vi "Start and Stop Continuous.vi"() -> (0 "x*y 3":dbl)   [LabVIEW 2010]
panel:
  out "Pitch Gauge (Degrees) 2":dbl(slide) scale=-90.0..90.0
  out "Roll Gauge (Degrees) 3":dbl(knob) scale=-180.0..180.0
  out "Roll Gauge (Degrees) 2":dbl(knob) scale=-180.0..180.0
  out "x*y 2":dbl
  out "x*y":dbl
  out "Command String":string
  in  "stop":bool
  in  "Stop Continuous":bool
  in  "Start":bool
  in  "Baud Rate":u32=115200
  in  "Serial Port":refnum<visa-resource-name>="COM1"
  out "Error Output":errorcluster
  out "Acceleration (G's)":dbl[](array[numeric])
  # "HOW TO USE\n\nSelect the port that your sensor is connected to, then click the \"Run\" arrow.  Click \"Start Continuous\" to start continuous mode and \"Stop Continuous\"  to stop continuous mode. Press STOP to stop vi and close port. The Acceleration and Angular Rate (0xC2 command) is displayed. \n\nFor USB sensors, use the Windows Device Manager to determine which COM port has been assigned to your sensor.  Your device will be listed as a  \"MicroStrain Virtual COM Port\".\n\nThe default BAUD rate is 115200 on all devices.  \n\nIf your device's port does not appear in the serial port control  then try quitting and relaunching LabVIEW."
  # "This example uses the 0xC4 command to start the 3DM-GX3 sending 0xC2 data packets continuously.   The data rate may be changed by using the Set Data Rate example."
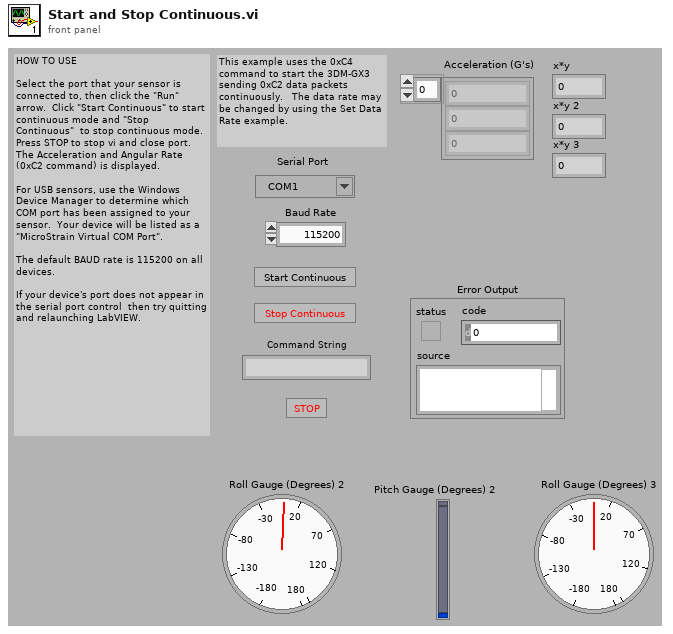
[diagram p1: front panel]
types:
  T1 = cluster{"Cmd/SOP Byte":string, "Header Size":u16, "Len":u16, "Chksum Start":u16, "Chksum End":i16, "InHdr":bool}[]
  T2 = cluster{"Command Byte":u8, "Acceleration Vector":cluster{sgl, sgl, sgl}, "Timer Ticks":u32, "Checksum":u16}
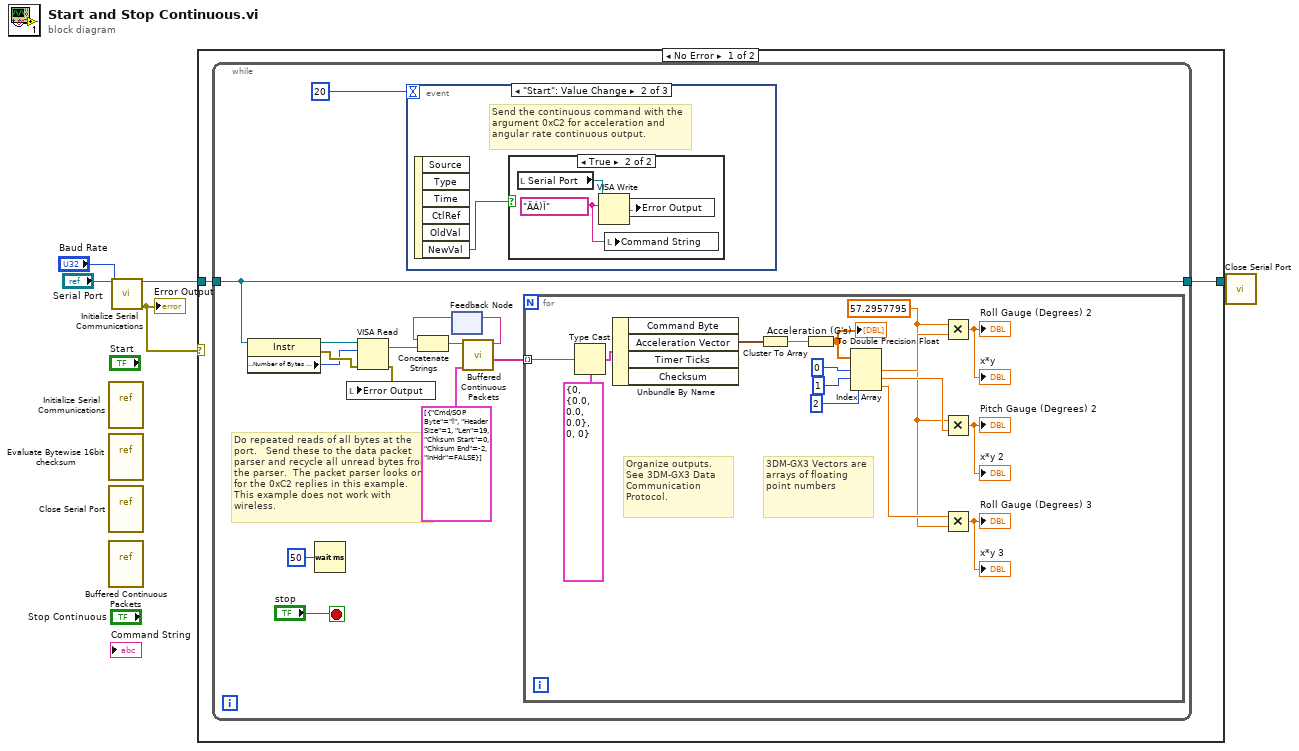
[diagram p0: block diagram]
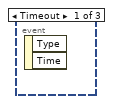
[diagram p2: hidden frame]
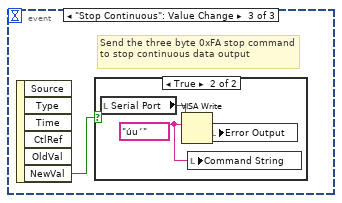
[diagram p4: hidden frame]
diagram:
  n1 = vi-ref "Initialize Serial Communications.vi"() -> ()  [unwired: 1 out]
  n2 = vi-ref "Evaluate Bytewise 16bit checksum.vi"() -> ()  [unwired: 1 out]
  n3 = vi-ref "Close Serial Port.vi"() -> ()  [unwired: 1 out]
  n4 = vi-ref "Buffered Continuous Packets.vi"() -> ()  [unwired: 1 out]
  n5 = call "Initialize Serial Communications.vi"("Serial Port"="Serial Port", "Baud Rate"="Baud Rate") -> ("Serial Port Out"=w3:refnum<visa-resource-name>, "error out"=w1:errorcluster)  [unwired: 12 in]
  "Error Output" <- w1
  n6 = case shown="No Error" w1 {
    tunnel: w3 -> [w7 w46]
    tunnel: [w6 w46] -> w2
    frame No Error {
      n7 = while {
        tunnel: w7 -> [w15]
        tunnel: [w15] -> w6
        stop <- "stop" stop-if-true
        # "Do repeated reads of all bytes at the port.   Send these to the data packet parser and recycle all unread bytes from the parser.  The packet parser looks only for the 0xC2 replies in this example.  This example does not work with wireless."
        n8 = property class="Instr"(reference=w15) -> (reference out=w18:refnum<visa-resource-name>, error out=w21:errorcluster, "Serial Settings:Number of Bytes at Serial Port"=w19:u32)  [unwired: 1 in]
        n9 = Wait (ms)(milliseconds to wait=u32 50) -> ()  [unwired: 1 out]
        n10 = VISA Read(VISA resource name=w18, byte count=w19, error in (no error)=w21) -> (read buffer=w20:string, error out=w14:errorcluster)  [unwired: 2 out]
        n11 = local write "Error Output"(w14) -> ()
        n12 = event shown="[1] \"Start\": Value Change" {
          selector: _ -> [_ _ _]
          dyn-events: _ -> [_ _ _]
          timeout: 20 -> [_ _ _]
          event Timeout {
            n13 = event-data() -> ()  [unwired: 1 in, 2 out]
          }
          event "Start": Value Change {
            # "Send the continuous command with the argument 0xC2 for acceleration and angular rate continuous output."
            n14 = event-data() -> ("NewVal"=w22:bool)  [unwired: 1 in, 5 out]
            n15 = case shown="True" w22 {
              frame False {
              }
              frame True {
                w23 = "ÄÁ)Î" ("write buffer")
                n16 = local read "Serial Port"() -> (w25:refnum<visa-resource-name>)
                n17 = VISA Write(VISA resource name=w25, write buffer=w23) -> (error out=w24:errorcluster)  [unwired: 1 in, 2 out]
                n18 = local write "Command String"(w23) -> ()
                n19 = local write "Error Output"(w24) -> ()
              }
            }
          }
          event "Stop Continuous": Value Change {
            # "Send the three byte 0xFA stop command to stop continuous data output"
            n20 = event-data() -> ("NewVal"=w26:bool)  [unwired: 1 in, 5 out]
            n21 = case shown="True" w26 {
              frame False {
              }
              frame True {
                w27 = "úu´" ("write buffer")
                n22 = local read "Serial Port"() -> (w29:refnum<visa-resource-name>)
                n23 = VISA Write(VISA resource name=w29, write buffer=w27) -> (error out=w28:errorcluster)  [unwired: 1 in, 2 out]
                n24 = local write "Command String"(w27) -> ()
                n25 = local write "Error Output"(w28) -> ()
              }
            }
          }
        }
        n26 = feedback #1() -> (w17:string)  [unwired: 1 in]
        n27 = Concatenate Strings(w17, w20) -> (w11:string)
        n28 = call "Buffered Continuous Packets.vi"("Input Buffer"=w11, "Packet definitions"=T1 [{"Cmd/SOP Byte"="Î", "Header Size"=1, "Len"=19, "Chksum Start"=0, "Chksum End"=-2, "InHdr"=FALSE}]) -> ("Remainder String"=w10:string, "Valid Records Found"=w9:string[])  [unwired: 4 in, 3 out]
        n29 = feedback-in #1(w10) -> ()
        n30 = for {
          tunnel: w9 -> [w41] mode=indexing
          w33 = 57.2957795 ("x")
          # "3DM-GX3 Vectors are arrays of floating point numbers"
          # "Organize outputs.  See 3DM-GX3 Data Communication Protocol."
          n31 = Type Cast(type=T2 {"Command Byte"=0, "Acceleration Vector"={0.0, 0.0, 0.0}, "Timer Ticks"=0, "Checksum"=0}, x=w41) -> (*(type *) &x=w44:T2)
          n32 = Unbundle By Name(w44) -> ("Acceleration Vector"=w43:cluster{sgl, sgl, sgl})  [unwired: 3 out]
          n33 = Cluster To Array(cluster=w43) -> (array=w42:sgl[])
          n34 = To Double Precision Float(number=w42) -> (double precision float=w40:dbl[])
          "Acceleration (G's)" <- w40
          n35 = Index Array(array=w40, index #1=0 ("index"), index #2=1 ("index"), index #3=2 ("index")) -> (element #1=w36:dbl, element #2=w35:dbl, element #3=w34:dbl)
          n36 = Multiply(x=w33, y=w36) -> (x*y=→"x*y" →"Roll Gauge (Degrees) 2":dbl)
          n37 = Multiply(x=w33, y=w35) -> (x*y=→"x*y 2" →"Pitch Gauge (Degrees) 2":dbl)
          n38 = Multiply(x=w34, y=w33) -> (x*y=→"x*y 3" →"Roll Gauge (Degrees) 3":dbl)
        }
      }
    }
    frame Error {
    }
  }
  n39 = call "Close Serial Port.vi"("Serial Port"=w2) -> ()  [unwired: 1 in, 1 out]
